vi "Write Array of Channel Control.vi"(10 "Array in":bool[](array[boolean]), 11 "Generic Data Logger.lvlib:Generic Data Logger Card.lvclass":refnum<class "Generic Data Logger Card.lvclass">) -> (3 "Generic Data Logger Card out":refnum<class "Generic Data Logger Card.lvclass">)   [LabVIEW 2013, in "Generic Data Logger.lvlib" / "Generic Data Logger Card.lvclass"]
uses:
  Generic Data Logger Card.lvclass
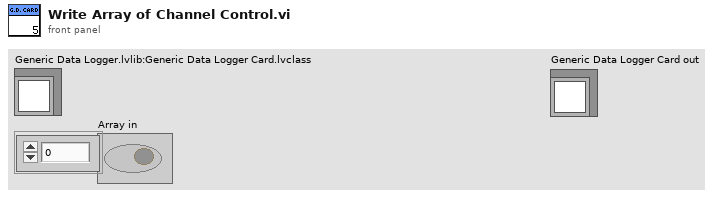
[diagram p1: front panel]
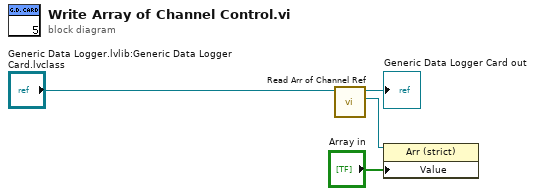
[diagram p0: block diagram]
diagram:
  n1 = call "Read Arr of Channel Ref.vi"("Generic Data Logger Card in"="Generic Data Logger.lvlib:Generic Data Logger Card.lvclass") -> ("Arr of Channel Ref"=w3:refnum<vi>, "Generic Data Logger Card out"=→"Generic Data Logger Card out":refnum<class "Generic Data Logger Card.lvclass">)  [unwired: 8 in, 1 out]
  n2 = property class="Arr (strict)"(reference=w3, "Value"="Array in") -> ()  [unwired: 1 in, 2 out]
